vi "Pixelated Image.vi"() -> ()   [LabVIEW 2019]
uses:
  <vilib>/FPGAPlugInAG/myRIO-1900/niLvFpga_Open_myRIO-1900.vi
  <vilib>/rvi/interface/common/dynamic/niFpgaDynamicAddResources.vi
  <vilib>/rvi/interface/nirviOpenFPGA/nirviOpenFPGA.xnode
  Collin's Project/FPGA Bitfiles/MRmecanum_FPGATarget_FPGAMainModified_TerasRobot_LKSN2021.lvbitx
panel:
  in  "Stop":bool
  out "Image Out":T1(plugin-control)
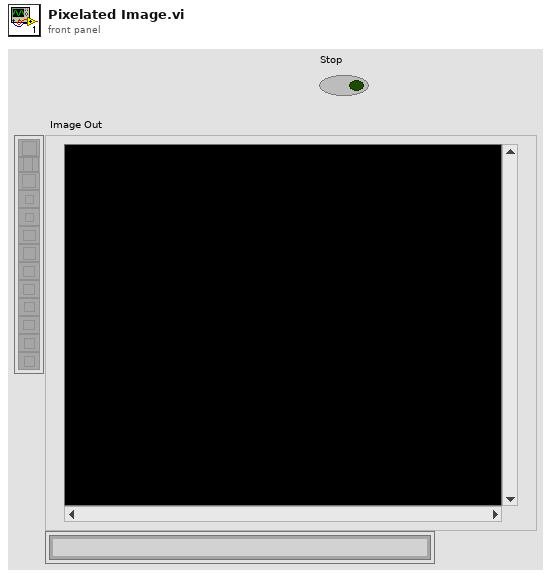
[diagram p1: front panel]
types:
  T1 = typedef "IMAQ Image.ctl" = refnum<image>
  T2 = enum16{"maju", "mundur", "kanan", "kiri", "atas kanan", "atas kiri", "bawah kanan", "bawah kiri", "putar kanan", "putar kiri"}
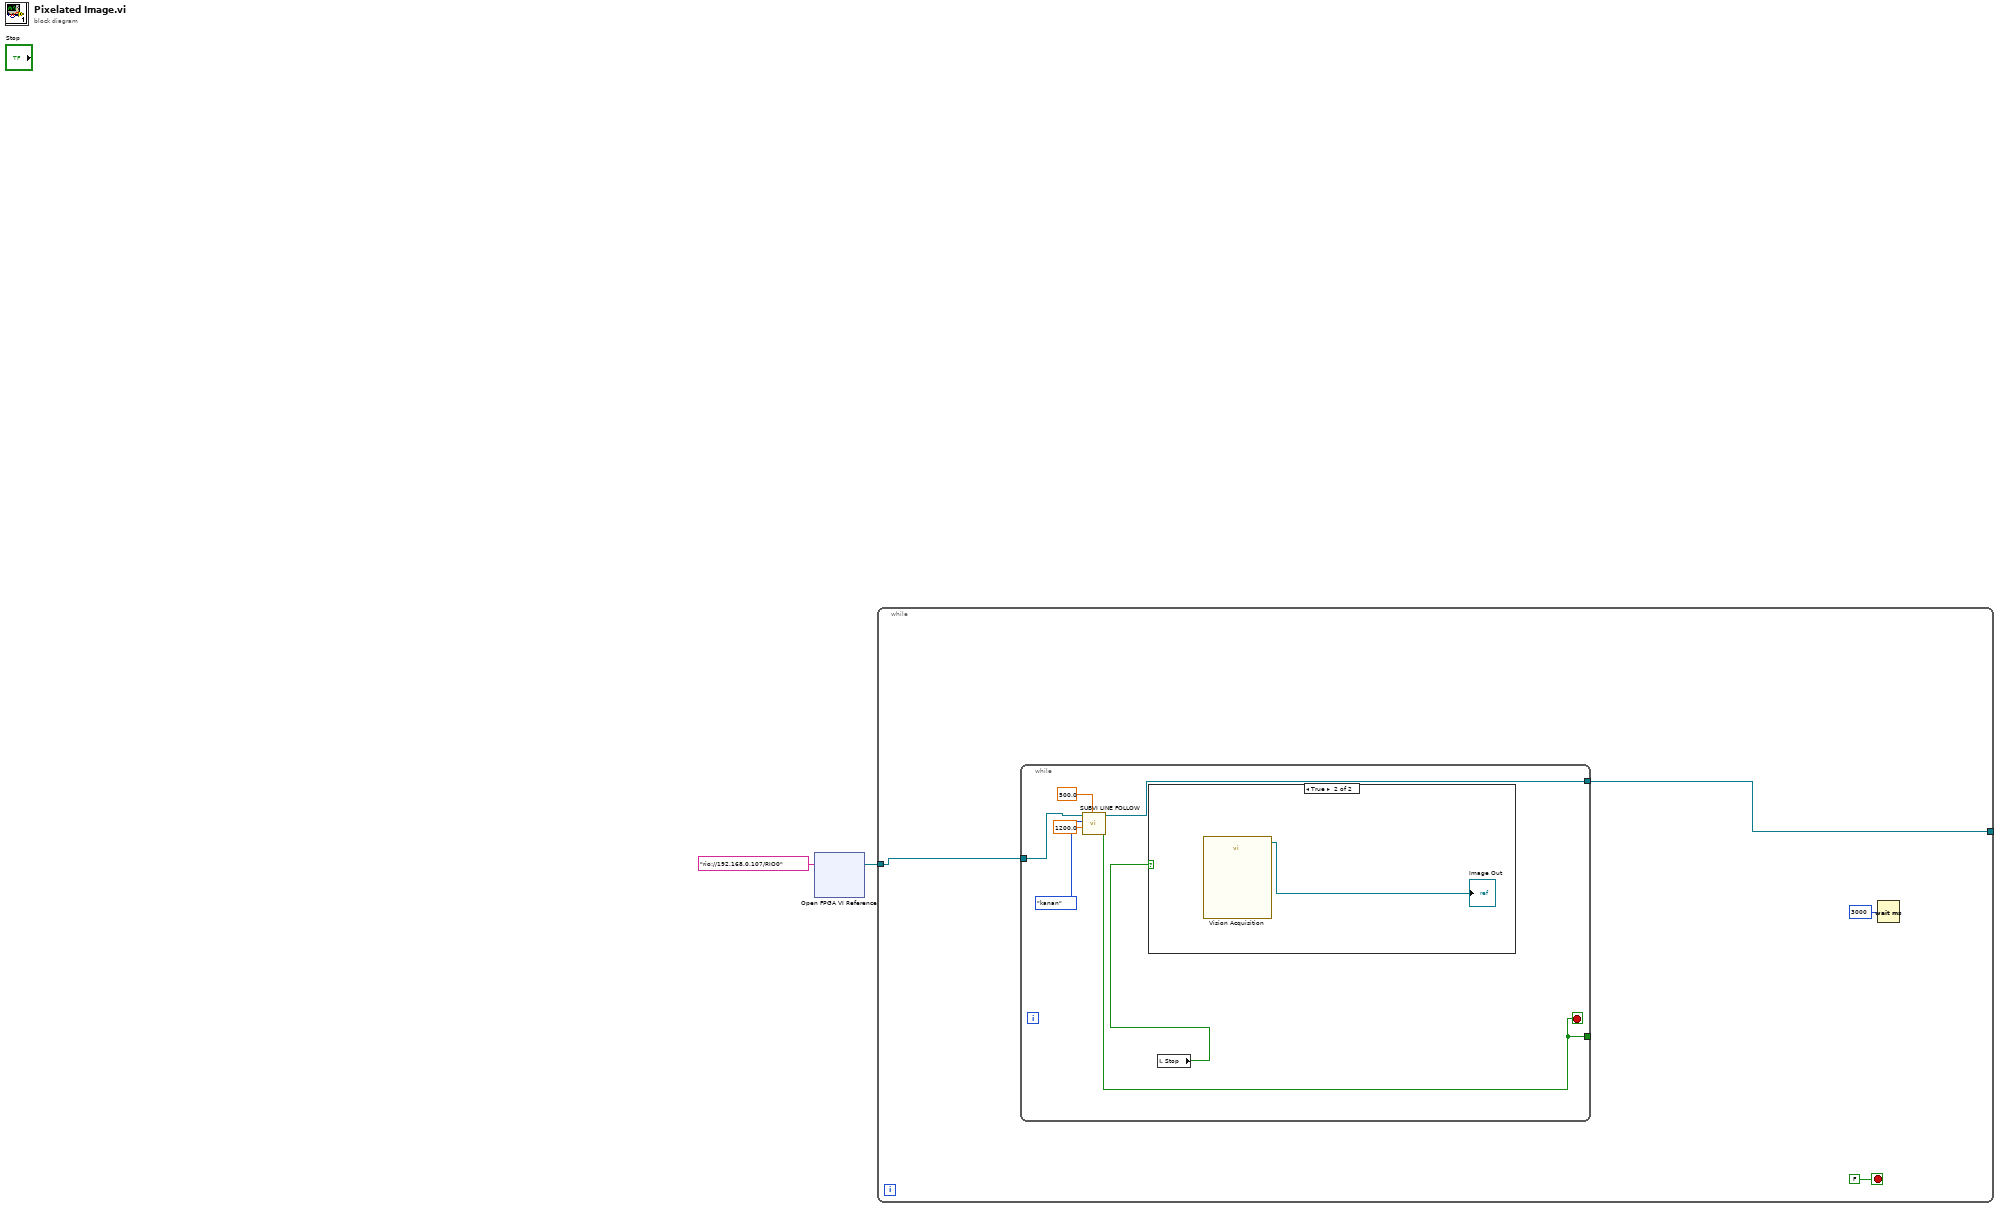
[diagram p0: block diagram]
diagram:
  n1 = xnode "Open FPGA VI Reference"("resource name"=tag "rio://192.168.0.107/RIO0") -> ("FPGA VI Reference Out"=w1:refnum<k20>)  [unwired: 1 in, 1 out]
  n2 = while {
    tunnel: [w5] -> _
    tunnel: w1 -> [w6]
    stop <- FALSE stop-if-true
    n3 = while {
      tunnel: w6 -> [w12]
      tunnel: [w11] -> w5
      tunnel: [w10] -> _
      stop <- w10 stop-if-true
      n4 = call "SUBVI LINE FOLLOW.vi"("Time"=500.0, "Value"=1200.0, "Move"=T2."kanan", "FPGA VI Reference Out 2"=w12) -> ("STOP?"=w10:bool, "FPGA VI Reference Out"=w11:refnum<k20>)  [unwired: 5 in, 1 out]
      n5 = local read "Stop"() -> (w13:bool)
      n6 = case shown="True" w13 {
        frame False {
        }
        frame True {
          n7 = call "Vision Acquisition"() -> ("Image Out"=→"Image Out":T1)  [unwired: 25 in, 2 out]
        }
      }
    }
    n8 = Wait (ms)(milliseconds to wait=u32 3000) -> ()  [unwired: 1 out]
  }
